vi "fgv_ledmatrix_config.vi"(7 "cmd":T2, 11 "data":T1={"ip"="", "data"="", "Port"="COM6", "time"=""}) -> (3 "data out":T1={"ip"="", "data"="", "Port"="COM6", "time"=""})   [LabVIEW 2019]
uses:
  Ctrl/cmd_common.ctl
  Ctrl/ledmatrix_data.ctl
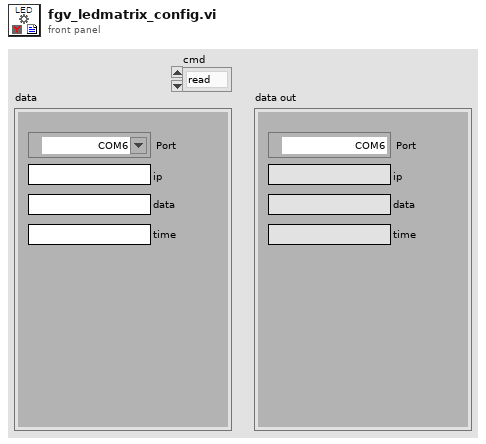
[diagram p1: front panel]
types:
  T1 = typedef "ledmatrix_data.ctl" = cluster{"ip":string, "data":string, "Port":refnum<visa-resource-name>, "time":string}
  T2 = typedef "cmd_common.ctl" = enum16{"read", "write"}
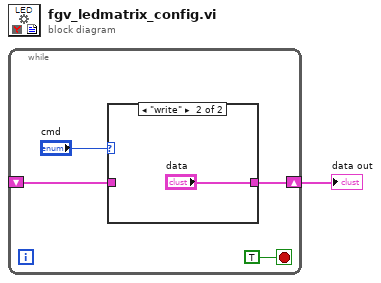
[diagram p0: block diagram]
diagram:
  n1 = while {
    shift-right: [w3] -> w1
    shift-left: _ -> [w2]
    stop <- TRUE stop-if-true
    n2 = case shown="\"write\"" "cmd" {
      tunnel: [w6 "data"] -> w3
      tunnel: w2 -> [w6 _]
      frame "read", Default {
      }
      frame "write" {
      }
    }
  }
  "data out" <- w1
